vi "Toggle Button.vi"(9 "button":bool) -> (1 "State":bool)   [LabVIEW 2019]
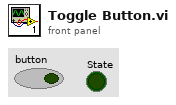
[diagram p1: front panel]
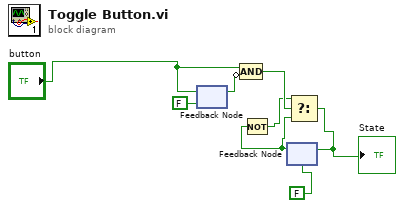
[diagram p0: block diagram]
diagram:
  n1 = feedback #1(FALSE ("Button 8")) -> (w8:bool)
  n2 = feedback-in #1("button") -> ()
  n3 = Compound Arithmetic op=AND("button", invert w8) -> (w6:bool)
  n4 = feedback #2(FALSE ("Button 8")) -> (w2:bool)
  n5 = Not(x=w2) -> (.not. x?=w3:bool)
  n6 = Select(t=w3, s=w6, f=w2) -> (s? t:f=w4:bool)
  "State" <- w4
  n7 = feedback-in #2(w4) -> ()
